vi "Init Reply.vi"(8 "error in (no error)":errorcluster, 11 "Mock Sift Proxy Server in":refnum<class "Mock Sift Proxy Server.lvclass">) -> (0 "error out":errorcluster, 3 "Mock Sift Proxy Server out":refnum<class "Mock Sift Proxy Server.lvclass">)   [LabVIEW 2024, in "Mock Sift Proxy Server.lvclass"]
uses:
  Mock Sift Proxy Server.lvclass
  Mock Sift Proxy Server.lvclass/Mock Sift Proxy Server.ctl
panel:
  out "Request":string
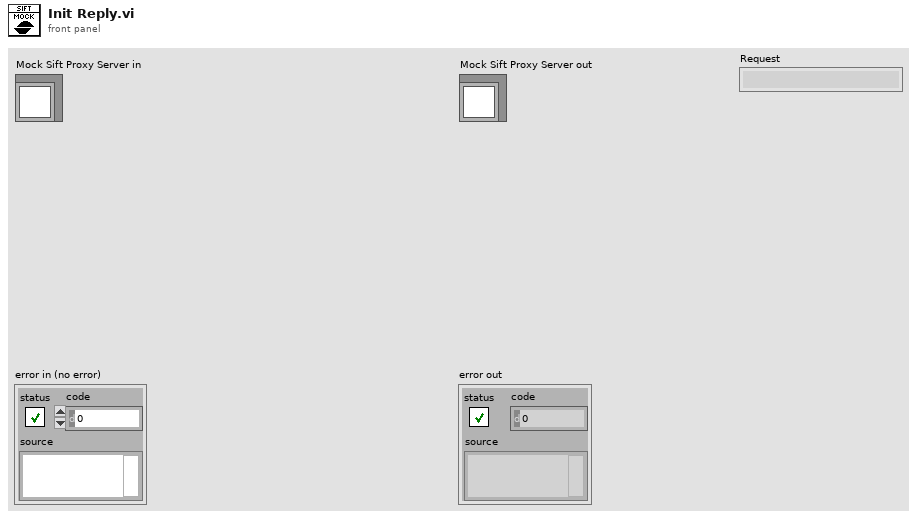
[diagram p1: front panel]
types:
  T1 = enum16{"Standard", "Buffered", "CRLF", "Immediate"}
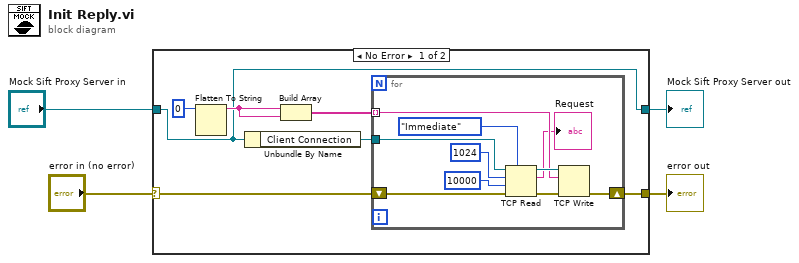
[diagram p0: block diagram]
diagram:
  n1 = case shown="No Error" "error in (no error)" {
    selector: "error in (no error)" -> [w6 w23]
    tunnel: [w5 w23] -> w3
    tunnel: [w8 w22] -> w1
    tunnel: "Mock Sift Proxy Server in" -> [w8 w22]
    frame No Error {
      n2 = Flatten To String(anything=u8 0) -> (data string=w10:string)  [unwired: 3 in, 2 out]
      n3 = Unbundle By Name(w8) -> ("Client Connection"=w7:refnum<k5>)
      n4 = Build Array(w10, w10) -> (w9:string[])
      n5 = for {
        tunnel: w9 -> [w18] mode=indexing
        tunnel: w7 -> [w17]
        shift-right: [w15] -> w5
        shift-left: w6 -> [w16]
        n6 = TCP Read(connection ID=w17, bytes to read=1024, error in (no error)=w16, 7:T1."Immediate" ("mode (standard)"), 9:10000 ("timeout ms (25000)")) -> (connection ID out=w21:refnum<k5>, data out=→"Request":string, error out=w20:errorcluster)
        n7 = TCP Write(connection ID=w21, data in=w18, error in (no error)=w20) -> (error out=w15:errorcluster)  [unwired: 1 in, 2 out]
      }
    }
    frame Error {
    }
  }
  "error out" <- w3
  "Mock Sift Proxy Server out" <- w1
